vi "Laps.vi"(11 "polar_pos":dbl[](array[numeric])) -> (3 "current_lap":dbl)   [LabVIEW 2012]
uses:
  <vilib>/Simulation/Implementation/Shared/SIMSCR Execution Mode.ctl
  <vilib>/Simulation/Scripting/Companion Diagram/SimConfigNode/SimParams.ctl
  <vilib>/Simulation/Scripting/Companion Diagram/SimConfigNode/_simSolvers.ctl
  <vilib>/Simulation/Param Hierarchy/Typedefs/SIMPH Param Control Actions.ctl
  <vilib>/Simulation/Implementation/Shared/NILVSim_FinalizeModel.vi
  <vilib>/Simulation/Utility/Implementation/NILVSim Memory.llb/NILVSim Memory (core).vi
  <vilib>/Simulation/Implementation/Shared/NILVSim_Manager.vi
  <vilib>/Simulation/Implementation/Shared/NILVSim_ParamChanged.vi
  <vilib>/Simulation/Implementation/Shared/SIM Bundle Sim Info.vi
  <vilib>/Simulation/Implementation/Shared/SIM SimErrorHandler.vi
  <vilib>/Simulation/Implementation/Shared/NILVSim_GetModelError.vi
  <vilib>/Utility/error.llb/Clear Errors.vi
  <vilib>/Simulation/Implementation/Shared/SIM Unbundle Sim Info.vi
  <vilib>/Simulation/Implementation/Shared/SIMSH Read Queue.vi
  <vilib>/Simulation/Implementation/Shared/NILVSim_Initialize.vi
  <vilib>/Simulation/Utility/Implementation/NILVSim Get Time and IsAcceptedStep.vi
  <vilib>/imath/engines/lvmath2/RunTimeEngine/ErrorHandling/NIMS_Finalize Error.vi
  <vilib>/imath/engines/lvmath2/RunTimeEngine/NodeEndStatement/NIMS_NodeEndStatement_Output.vi
  <instcachedir>/0/NIMS_NodeEndStatement_Output_53EC0D466D134D7ABD903AC30B43404B.lvgen/NIMS_NodeEndStatement_Output_53EC0D466D134D7ABD903AC30B43404B_001.vi
  <vilib>/imath/engines/lvmath2/RunTimeEngine/CommandStatement/NIMS_CommandStatement_MaskErr.vi
  <vilib>/imath/engines/lvmath2/RunTimeEngine/CommandStatement/MC_CommandStatement_break.vi
  <vilib>/Simulation/Scripting/Companion Diagram/SimConfigNode/SimDog.xnode
  <vilib>/Simulation/Implementation/XNodeFramework/SimXNode/SimX.xnode
  <vilib>/Simulation/Implementation/Shared/NI_SIM_Implementation.lvlib
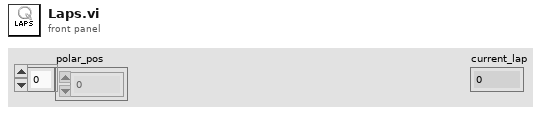
[diagram p1: front panel]
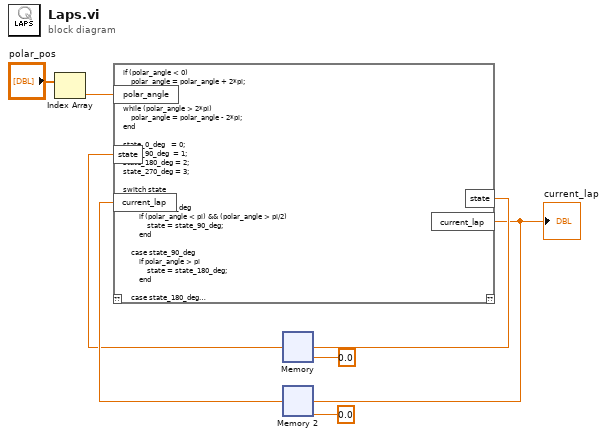
[diagram p0: block diagram]
diagram:
  n1 = Index Array(array="polar_pos") -> (element=w5:dbl)  [unwired: 1 in]
  n2 = mathscript code="if (polar_angle < 0)\n    polar_angle = polar_angle + 2*pi;\nend\n\nwhile (polar_angle > 2*pi)\n    polar_angle = polar_angle - 2*pi;\nend\n\nstate_0_deg   = 0;\nstate_90_deg  = 1;\nstate_180_deg = 2;\nstate_270_deg = 3;\n\nswitch state\n    \n    case state_0_deg\n        if (polar_angle < pi) && (polar_angle > pi/2)\n            state = state_90_deg;\n        end\n        \n    case state_90_deg\n        if polar_angle > pi\n            state = state_180_deg;\n        end\n\n    case state_180_deg\n        if polar_angle > pi*3/2\n            state = state_270_deg;\n        end\n        \n    case state_270_deg\n        if (polar_angle < pi*3/2) && (polar_angle > pi)\n           state = state_180_deg; \n        elseif (polar_angle > 0) && (polar_angle < pi/2)\n           state = state_0_deg;\n           current_lap = current_lap + 1;\n        end    \nend\n\nLap = current_lap;\ncurrent_state = state;"("polar_angle"=w5, "state"=w6, "current_lap"=w7) -> ("state"=w2:dbl, "current_lap"=w1:dbl)  [unwired: 1 in, 1 out]
  "current_lap" <- w1
  n3 = xnode "Memory"("input"=w2, "initial value"=0.0) -> ("output"=w6:dbl)  [unwired: 4 in]
  n4 = xnode "Memory 2"("input"=w1, "initial value"=0.0 ("initial value 2")) -> ("output"=w7:dbl)  [unwired: 4 in]
